vi "Load Plugin Child Class by Name.vi"(8 "error in (no error)":errorcluster, 9 "Plugin Directory Path":path=path "../Plugins", 10 "Plugin Child Class Name":string, 11 "Base Class":refnum<class>) -> (0 "error out":errorcluster, 3 "Plugin Child Class":refnum<class>)   [LabVIEW 2016, in "SLL Class.lvlib"]
doc: "Load a child class plugin by name. Supports normal classes, classes within PPLs and classes within EXEs.\n\nThe plugin directory path is optional and can be either absolute path or relative path. If relative, the path would be taken relative to the base class directory. By default, the plugins directory is assumed to be present parallel to the base class directory, like below.\n\nBase\nPlugins/Plugin 1/Plugin 1.lvclass\nPlugins/Plugin 2/Plugin 2.lvlibp"
uses:
  SLL Class.lvlib
  SLL File IO/SLL File IO.lvlib
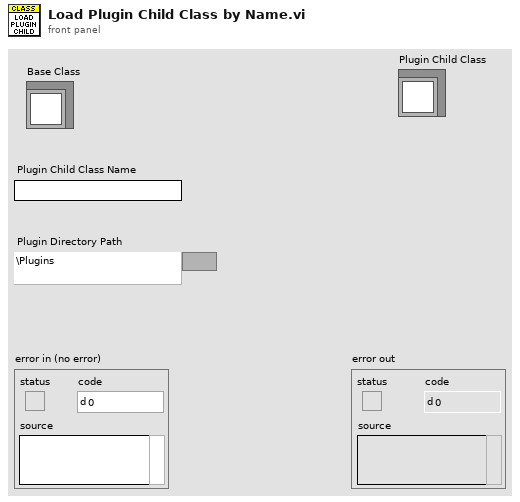
[diagram p1: front panel]
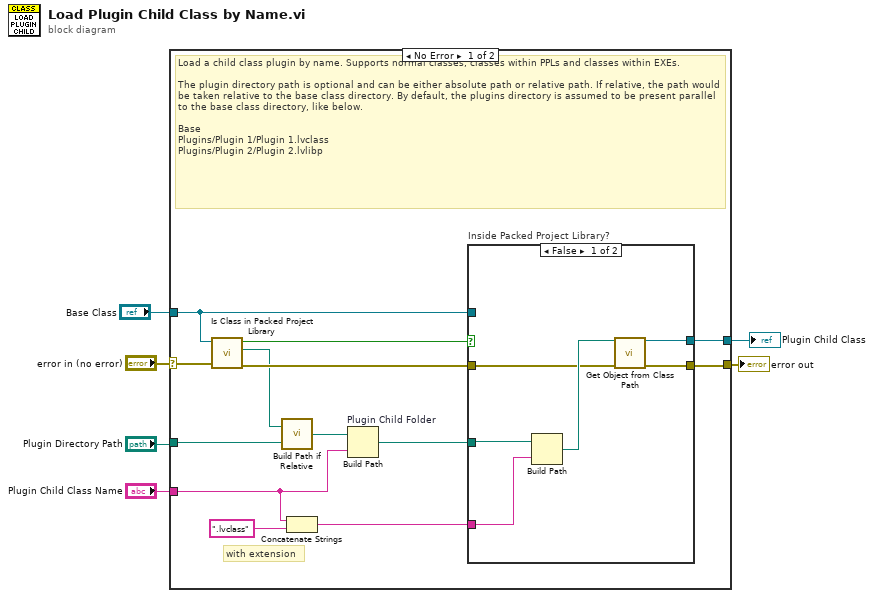
[diagram p0: block diagram]
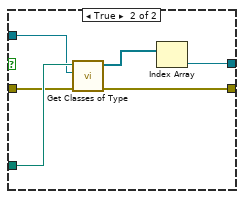
[diagram p2: hidden frame]
diagram:
  n1 = case shown="No Error" "error in (no error)" {
    selector: "error in (no error)" -> [w17 w32]
    tunnel: [w16 w32] -> w5
    tunnel: "Base Class" -> [w10 _]
    tunnel: "Plugin Directory Path" -> [w8 _]
    tunnel: "Plugin Child Class Name" -> [w12 _]
    tunnel: [w15 _] -> w1
    frame No Error {
      # "with extension"
      # "Load a child class plugin by name. Supports normal classes, classes within PPLs and classes within EXEs.\n\nThe plugin directory path is optional and can be either absolute path or relative path. If relative, the path would be taken relative to the base class directory. By default, the plugins directory is assumed to be present parallel to the base class directory, like below.\n\nBase\nPlugins/Plugin 1/Plugin 1.lvclass\nPlugins/Plugin 2/Plugin 2.lvlibp"
      n2 = call "Is Class in Packed Project Library.vi"("error in (no error)"=w17, "Class"=w10) -> ("error out"=w18:errorcluster, "Class Directory"=w9:path, "In Packed Project Library?"=w19:bool)  [unwired: 6 in, 1 out]
      n3 = call "Build Path if Relative.vi"("Relative or Absolute Path"=w8, "Base Path"=w9) -> ("Path Out"=w7:path)
      n4 = Concatenate Strings(w12, ".lvclass" ("string")) -> (w13:string)
      n5 = Build Path "Plugin Child Folder"(base path=w7, name or relative path=w12) -> (appended path=w11:path)
      n6 = case "Inside Packed Project Library?" shown="False" w19 {
        tunnel: w18 -> [w24 w29]
        tunnel: [w23 w26] -> w16
        tunnel: [w22 w27] -> w15
        tunnel: w13 -> [w21 _]
        tunnel: w11 -> [w20 w31]
        tunnel: w10 -> [_ w30]
        frame False {
          n7 = Build Path(base path=w20, name or relative path=w21) -> (appended path=w25:path)
          n8 = call "Get Object from Class Path.vi"("LabVIEW Class Path"=w25, "error in (no error)"=w24) -> ("Object"=w22:refnum<class>, "error out"=w23:errorcluster)  [unwired: 12 in]
        }
        frame True {
          n9 = call "Get Classes of Type.vi"("error in (no error)"=w29, "Class Type"=w30, "Directory Path"=w31) -> ("error out"=w26:errorcluster, "Classes[]"=w28:refnum<class>[])  [unwired: 7 in]
          n10 = Index Array(array=w28) -> (element=w27:refnum<class>)  [unwired: 1 in]
        }
      }
    }
    frame Error {
    }
  }
  "error out" <- w5
  "Plugin Child Class" <- w1
